vi "LoadMPCMatrix_singleAxis_variableN.vi"(8 "nuN_mpc":u16, 9 "Ns+1":u16, 10 "FIFO Timeout\nIn":bool) -> (0 "FIFO Matrix Timeout":bool, 3 "error out":errorcluster)   [LabVIEW 2017]
uses:
  <vilib>/rvi/interface/RandomDataEmulation/niFpgaRandomDataHandleErrors.vi
  <vilib>/rvi/DataTransferAndStorage/Container/XNode/niFpgaContainer.xnode
  <vilib>/rvi/interface/RandomDataEmulation/nirviRandomDataFpgaReadWriteTemplate.vi
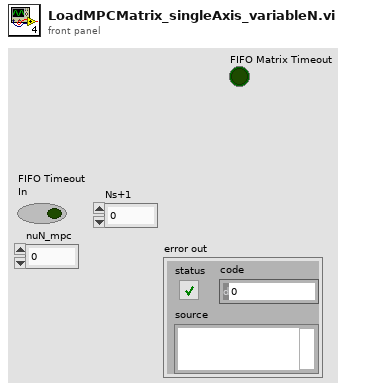
[diagram p1: front panel]
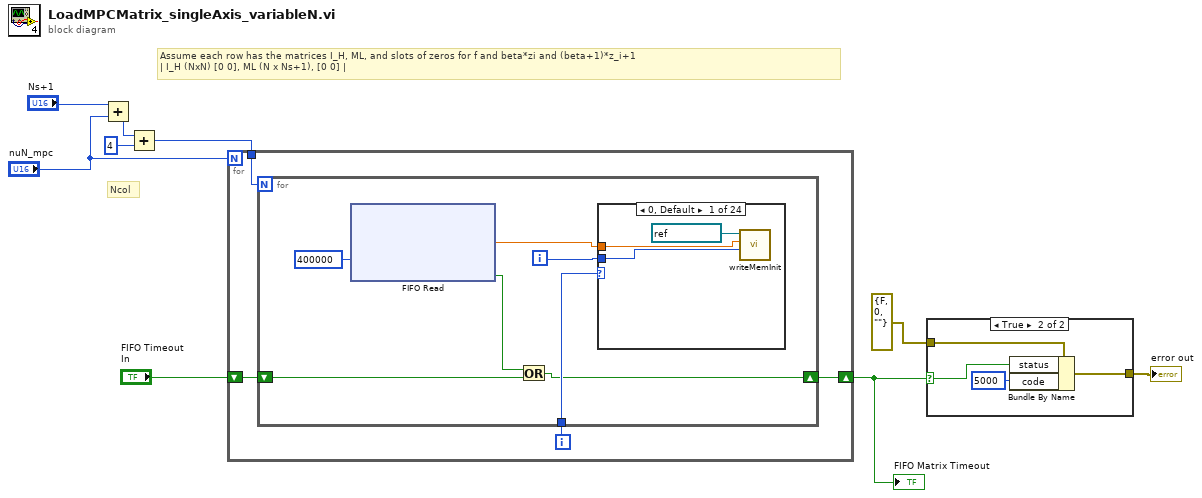
[diagram p0: block diagram]
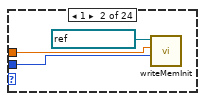
[diagram p2: hidden frame]
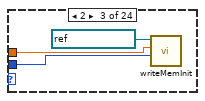
[diagram p3: hidden frame]
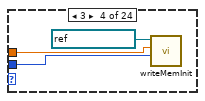
[diagram p4: hidden frame]
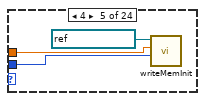
[diagram p5: hidden frame]
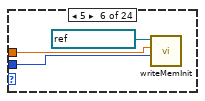
[diagram p6: hidden frame]
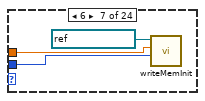
[diagram p7: hidden frame]
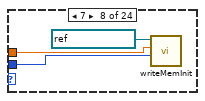
[diagram p8: hidden frame]
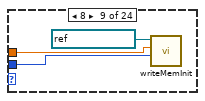
[diagram p9: hidden frame]
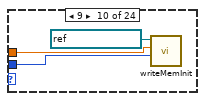
[diagram p10: hidden frame]
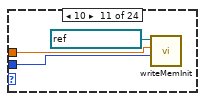
[diagram p11: hidden frame]
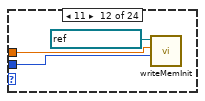
[diagram p12: hidden frame]
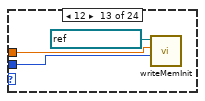
[diagram p13: hidden frame]
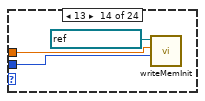
[diagram p14: hidden frame]
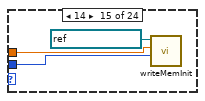
[diagram p15: hidden frame]
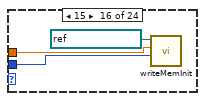
[diagram p16: hidden frame]
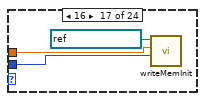
[diagram p17: hidden frame]
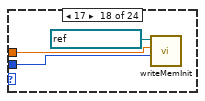
[diagram p18: hidden frame]
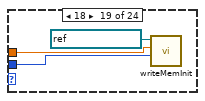
[diagram p19: hidden frame]
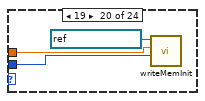
[diagram p20: hidden frame]
diagram:
  # "Ncol"
  # "Assume each row has the matrices I_H, ML, and slots of zeros for f and beta*zi and (beta+1)*z_i+1\n| I_H (NxN) [0 0], ML (N x Ns+1), [0 0] |"
  n1 = Add(x="Ns+1", y="nuN_mpc") -> (x+y=w7:u16)
  n2 = Add(x=w7, y=u16 4) -> (x+y=w5:u16)
  n3 = for {
    N: "nuN_mpc" -> [_]
    tunnel: w5 -> [w13]
    shift-right: [w10] -> w3
    shift-left: "FIFO Timeout\nIn" -> [w11]
    i -> [w12]
    n4 = for {
      N: w13 -> [_]
      tunnel: w12 -> [w17]
      shift-right: [w14] -> w10
      shift-left: w11 -> [w15]
      i -> [w19]
      n5 = xnode ("FIFO Read")("Timeout"=400000) -> ("Element"=w18:sgl, "Timed Out?"=w16:bool)  [unwired: 1 in, 1 out]
      n6 = Or(x=w16, y=w15) -> (x .or. y?=w14:bool)
      n7 = case shown="0, Default" w17 {
        tunnel: w18 -> [w22 w25 w28 w31 w34 w37 w40 w43 w46 w49 w52 w55 w58 w61 w64 w67 w70 w73 w76 w79 w82 w85 w88 w91]
        tunnel: w19 -> [w21 w24 w27 w30 w33 w36 w39 w42 w45 w48 w51 w54 w57 w60 w63 w66 w69 w72 w75 w78 w81 w84 w87 w90]
        frame 0, Default {
          n8 = call "writeMemInit.vi"("address"=w21, "data"=w22, "Memory"=refnum<k21> "Memory") -> ()  [unwired: 9 in]
        }
        frame 1 {
          n9 = call "writeMemInit.vi"("address"=w24, "data"=w25, "Memory"=refnum<k21> "Memory 2") -> ()  [unwired: 9 in]
        }
        frame 2 {
          n10 = call "writeMemInit.vi"("address"=w27, "data"=w28, "Memory"=refnum<k21> "Memory 3") -> ()  [unwired: 9 in]
        }
        frame 3 {
          n11 = call "writeMemInit.vi"("address"=w30, "data"=w31, "Memory"=refnum<k21> "Memory 4") -> ()  [unwired: 9 in]
        }
        frame 4 {
          n12 = call "writeMemInit.vi"("address"=w33, "data"=w34, "Memory"=refnum<k21> "Memory 5") -> ()  [unwired: 9 in]
        }
        frame 5 {
          n13 = call "writeMemInit.vi"("address"=w36, "data"=w37, "Memory"=refnum<k21> "Memory 6") -> ()  [unwired: 9 in]
        }
        frame 6 {
          n14 = call "writeMemInit.vi"("address"=w39, "data"=w40, "Memory"=refnum<k21> "Memory 7") -> ()  [unwired: 9 in]
        }
        frame 7 {
          n15 = call "writeMemInit.vi"("address"=w42, "data"=w43, "Memory"=refnum<k21> "Memory 8") -> ()  [unwired: 9 in]
        }
        frame 8 {
          n16 = call "writeMemInit.vi"("address"=w45, "data"=w46, "Memory"=refnum<k21> "Memory 9") -> ()  [unwired: 9 in]
        }
        frame 9 {
          n17 = call "writeMemInit.vi"("address"=w48, "data"=w49, "Memory"=refnum<k21> "Memory 10") -> ()  [unwired: 9 in]
        }
        frame 10 {
          n18 = call "writeMemInit.vi"("address"=w51, "data"=w52, "Memory"=refnum<k21> "Memory 11") -> ()  [unwired: 9 in]
        }
        frame 11 {
          n19 = call "writeMemInit.vi"("address"=w54, "data"=w55, "Memory"=refnum<k21> "Memory 12") -> ()  [unwired: 9 in]
        }
        frame 12 {
          n20 = call "writeMemInit.vi"("address"=w57, "data"=w58, "Memory"=refnum<k21> "Memory 13") -> ()  [unwired: 9 in]
        }
        frame 13 {
          n21 = call "writeMemInit.vi"("address"=w60, "data"=w61, "Memory"=refnum<k21> "Memory 14") -> ()  [unwired: 9 in]
        }
        frame 14 {
          n22 = call "writeMemInit.vi"("address"=w63, "data"=w64, "Memory"=refnum<k21> "Memory 15") -> ()  [unwired: 9 in]
        }
        frame 15 {
          n23 = call "writeMemInit.vi"("address"=w66, "data"=w67, "Memory"=refnum<k21> "Memory 16") -> ()  [unwired: 9 in]
        }
        frame 16 {
          n24 = call "writeMemInit.vi"("address"=w69, "data"=w70, "Memory"=refnum<k21> "Memory 17") -> ()  [unwired: 9 in]
        }
        frame 17 {
          n25 = call "writeMemInit.vi"("address"=w72, "data"=w73, "Memory"=refnum<k21> "Memory 18") -> ()  [unwired: 9 in]
        }
        frame 18 {
          n26 = call "writeMemInit.vi"("address"=w75, "data"=w76, "Memory"=refnum<k21> "Memory 19") -> ()  [unwired: 9 in]
        }
        frame 19 {
          n27 = call "writeMemInit.vi"("address"=w78, "data"=w79, "Memory"=refnum<k21> "Memory 20") -> ()  [unwired: 9 in]
        }
        frame 20 {
          n28 = call "writeMemInit.vi"("address"=w81, "data"=w82, "Memory"=refnum<k21> "Memory 21") -> ()  [unwired: 9 in]
        }
        frame 21 {
          # "Cant pull the write op\noutside, otherwise LV\ncomplains of a dynamic\nrefnum."
          n29 = call "writeMemInit.vi"("address"=w84, "data"=w85, "Memory"=refnum<k21> "Memory 22") -> ()  [unwired: 9 in]
        }
        frame 22 {
          n30 = call "writeMemInit.vi"("address"=w87, "data"=w88, "Memory"=refnum<k21> "Memory 23") -> ()  [unwired: 9 in]
        }
        frame 23 {
          n31 = call "writeMemInit.vi"("address"=w90, "data"=w91, "Memory"=refnum<k21> "Memory 24") -> ()  [unwired: 9 in]
        }
      }
    }
  }
  "FIFO Matrix Timeout" <- w3
  n32 = case shown="True" w3 {
    selector: w3 -> [_ w96]
    tunnel: errorcluster {"status"=FALSE, "code"=0, "source"=""} ("error in") -> [w93 w97]
    tunnel: [w93 w95] -> w9
    frame False {
    }
    frame True {
      n33 = Bundle By Name(cluster=w97, "status"=w96, "code"=5000) -> (w95:errorcluster)
    }
  }
  "error out" <- w9
